vi "Call_C.vi"(8 "error in (no error)":errorcluster, 11 "working directory":path=path "") -> (0 "error out 2":errorcluster, 1 "standard output":string, 2 "Traces":string)   [LabVIEW 2023]
panel:
  out "stripped path 3":path
  out "name 3":string
  out "return code":i32
  out "standard error":string
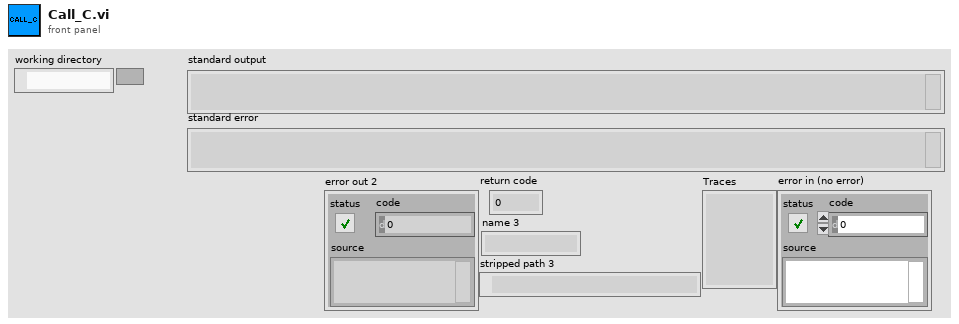
[diagram p1: front panel]
types:
  T1 = cluster{bool, "return code":i32, "standard error":string}
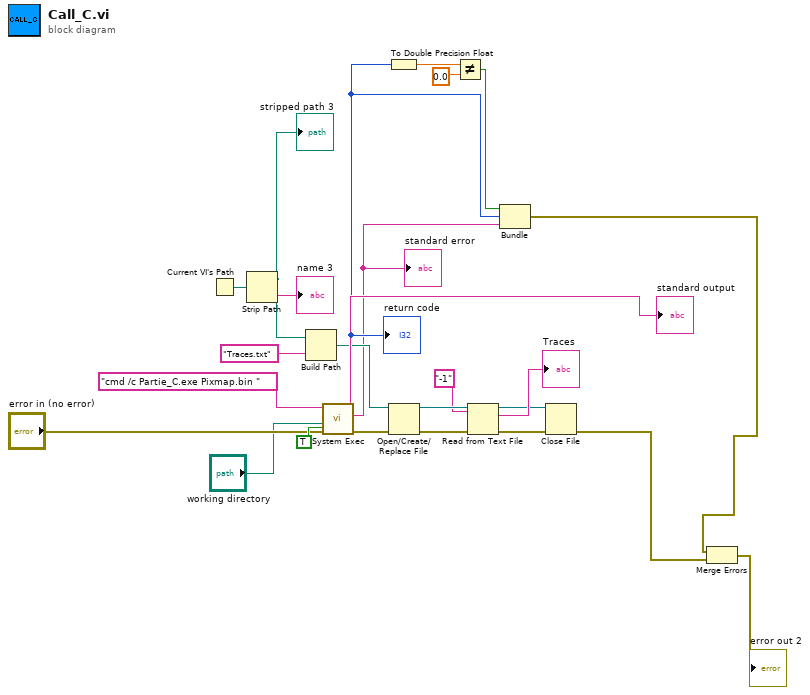
[diagram p0: block diagram]
diagram:
  n1 = Current VI's Path() -> (path=w22:path)
  n2 = Strip Path(path=w22) -> (stripped path=w19:path, name=→"name 3":string)
  "stripped path 3" <- w19
  n3 = Build Path(base path=w19, name or relative path="Traces.txt") -> (appended path=w18:path)
  n4 = call <vilib>:"System Exec.vi"("run minimized? (F)"=TRUE, "error in (no error)"="error in (no error)", "working directory"="working directory", "command line"="cmd /c Partie_C.exe Pixmap.bin ") -> ("error out"=w13:errorcluster, "return code"=w8:i32, "standard error"=w7:string, "standard output"=→"standard output":string)  [unwired: 4 in]
  "standard error" <- w7
  "return code" <- w8
  n5 = To Double Precision Float(number=w8) -> (double precision float=w10:dbl)
  n6 = Open/Create/Replace File(file path (use dialog)=w18, error in=w13) -> (refnum out=w17:refnum<file>, error out=w15:errorcluster)  [unwired: 4 in, 1 out]
  n7 = Not Equal?(x=w10, y=0.0) -> (x != y?=w6:bool)
  n8 = Read from Text File(prompt (Open existing file)="-1", file (use dialog)=w17, error in=w15) -> (refnum out=w11:refnum<file>, text=→"Traces":string, error out=w14:errorcluster)  [unwired: 1 in, 1 out]
  n9 = Bundle(w6, "return code"=w8, "standard error"=w7) -> (w2:T1)  [unwired: 1 in]
  n10 = Close File(refnum=w11, error in=w14) -> (error out=w3:errorcluster)  [unwired: 1 out]
  n11 = Merge Errors(w2, w3) -> (→"error out 2":errorcluster)
